vi "GasflaschenHeader.vi"() -> (2 "Trennlinie":string[](array[string]), 3 "Header":string[](array[string])=["Name of Gas", "Number (Cylinder)", "Batch", "Volume", "Date of Production", "Expiration Date", "Carrier Gas", "Gas 1", "Nominal", "Real", "Unit", "Accuracy %", "Gas 2", "Nominal", "Real", "Unit", "Accuracy %", "Gas 3", "Nominal", "Real", "Unit", "Accuracy %", "Gas 4", "Nominal", "Real", "Unit", "Accuracy %", "Gas 5", "Nominal", "Real", "Unit", "Accuracy %"])   [LabVIEW 2020, in "System Einstellungen V2.lvlib"]
uses:
  System Einstellungen V2.lvlib
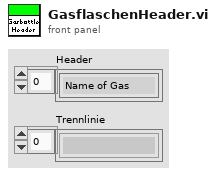
[diagram p1: front panel]
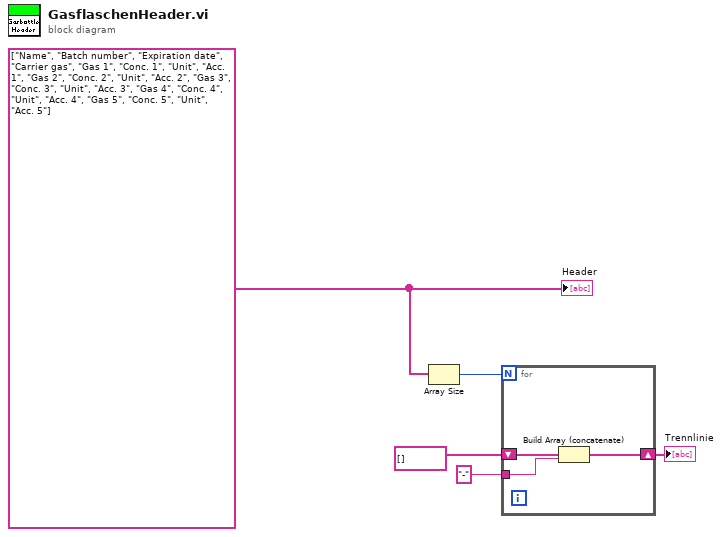
[diagram p0: block diagram]
diagram:
  w1 = string[] ["Name", "Batch number", "Expiration date", "Carrier gas", "Gas 1", "Conc. 1", "Unit", "Acc. 1", "Gas 2", "Conc. 2", "Unit", "Acc. 2", "Gas 3", "Conc. 3", "Unit", "Acc. 3", "Gas 4", "Conc. 4", "Unit", "Acc. 4", "Gas 5", "Conc. 5", "Unit", "Acc. 5"]
  n1 = Array Size(array=w1) -> (size(s)=w5:i32)
  n2 = for {
    N: w5 -> [_]
    tunnel: "-" -> [w8]
    shift-right: [w7] -> w2
    shift-left: string[] [] -> [w6]
    n3 = Build Array (concatenate)(w6, w8) -> (w7:string[])
  }
  "Trennlinie" <- w2
  "Header" <- w1
